vi "Get Scalar Datatypes and Refs.vi"(6 "Item Ref in":T1 format="%.0x", 8 "error in (no error)":errorcluster, 9 "Registers":T2[](array[typedef]) {"Register"."Data Type" format="%.0x"}, 10 "Data":dbl[](array[numeric]), 11 "Refs":T1[](array[typedef]) format="%.0x") -> (0 "error out":errorcluster, 1 "Registers out":T2[](array[typedef]) {"Register"."Data Type" format="%.0x"}, 2 "Data out":dbl[](array[numeric]), 3 "Refs out":T1[](array[typedef]) format="%.0x")   [LabVIEW 2018, in "FPGA Addon System Explorer.lvlib"]
uses:
  FPGA Addon System Explorer.lvlib
  Addon Shared/Types/Compiled.RegisterSettings.ctl
  Addon Shared/Types/Scalar Type.ctl
  Addon Shared/Types/Register Information.ctl
  Addon Shared/Types/FPGA Addon Data Type.ctl
  <vilib>/NI Veristand/Custom Device API/Custom Device Item Ref.ctl
  Addon Shared/Types/FG Action.ctl
  Addon Shared/SubVIs/Constants.vi
  <vilib>/NI/NI VeriStand Advanced SysDef API/SysDef API/SysDef.Property.Get.vi
  <vilib>/NI/NI VeriStand Advanced SysDef API/_SubVIs/SysDef.Property.Get.Variant.vi
  <vilib>/NI/NI VeriStand Advanced SysDef API/SysDef API/SysDef.Property.Set.vi
  <vilib>/NI/NI VeriStand Advanced SysDef API/_SubVIs/SysDef.Property.Set.Variant.vi
  <vilib>/NI Veristand/Custom Device API/Get Item Property (String).vi
  <vilib>/NI Veristand/Custom Device API/Custom Device API.lvlib
  Addon Shared/FPGA Addon Shared.lvlib
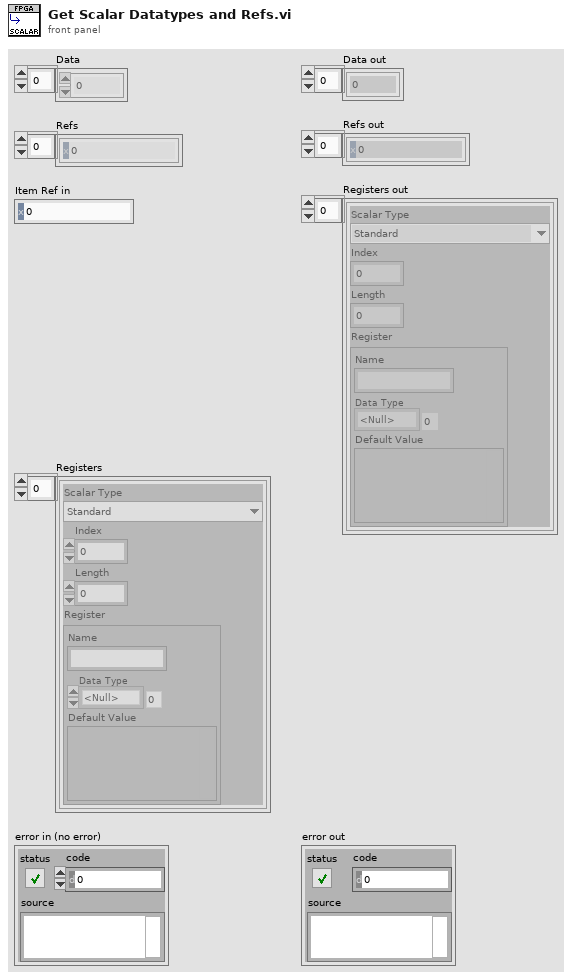
[diagram p1: front panel]
types:
  T1 = typedef "Custom Device API.lvlib/Custom Device Item Ref.ctl" = u64
  T2 = typedef "FPGA Addon Shared.lvlib/Compiled.RegisterSettings.ctl" = cluster{"Scalar Type":T3, "Index":i32, "Length":i32, "Register":T4}
  T3 = typedef "FPGA Addon Shared.lvlib/Scalar Type.ctl" = enum16{"Standard", "Bitpacked"}
  T4 = typedef "FPGA Addon Shared.lvlib/Register Information.ctl" = cluster{"Name":string, "Data Type":T5, "Default Value":variant}
  T5 = typedef "FPGA Addon Shared.lvlib/FPGA Addon Data Type.ctl" = enum8{"<Null>", "I8", "I16", "I32", "I64", "U8", "U16", "U32", "U64", "SGL", "Boolean", "Analog PWM In Settings", "Analog PWM In", "Digital PWM In Settings", "Digital PWM In", "Digital PWM Out", "Sine Out", "FXP", "FXP+/-24.5", "FXP+/-16.5", "FXP+/-32.8", "FXP+/-64.32", "FXP+/-16.7", "FXP+/-20.5", "FXP+/-27.5", "FXP+/-32.16", "FXP+16.3", "FXP+18.3", "Digital Static In", "Digital Static Out", "Digital Static In Settings", "Digital WSS Out", "Quad Encoder Settings", "Quad Encoder In", "Group"}
  T6 = typedef "FPGA Addon Shared.lvlib/FG Action.ctl" = enum8{"GET", "SET"}
  T7 = typedef "Custom Device API.lvlib/Custom Device Item Info.ctl" = cluster{"Name":string, "Is Channel":bool, "GUID":string, "Is Waveform":bool}
  T8 = typedef "Custom Device API.lvlib/Custom Device Channel.ctl" = cluster{"Type":T9, "Units":string, "Default Value":dbl, "Faultable":bool, "Scalable":bool}
  T9 = typedef "Custom Device API.lvlib/Custom Device Channel Type.ctl" = enum16{"Input", "Output"}
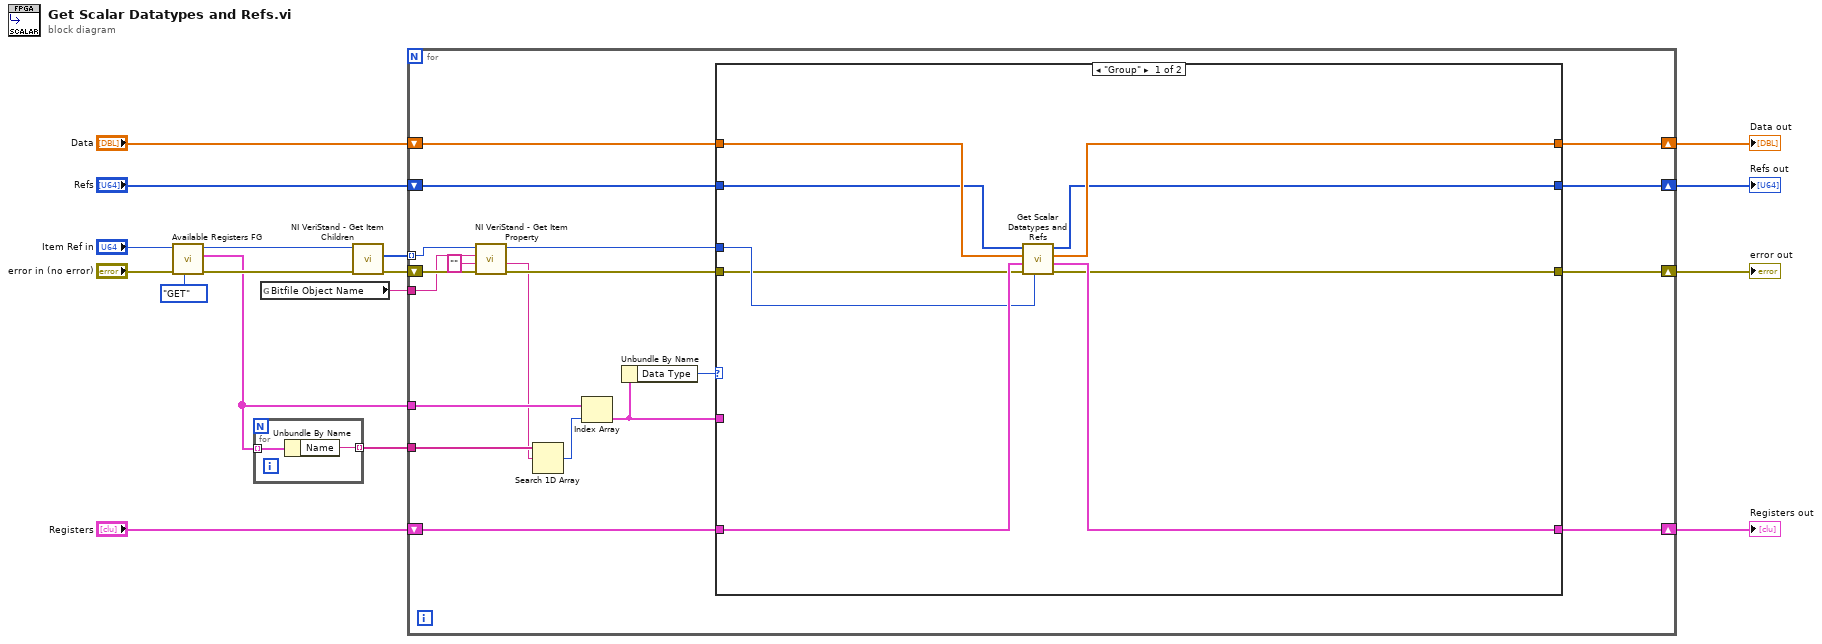
[diagram p0: block diagram]
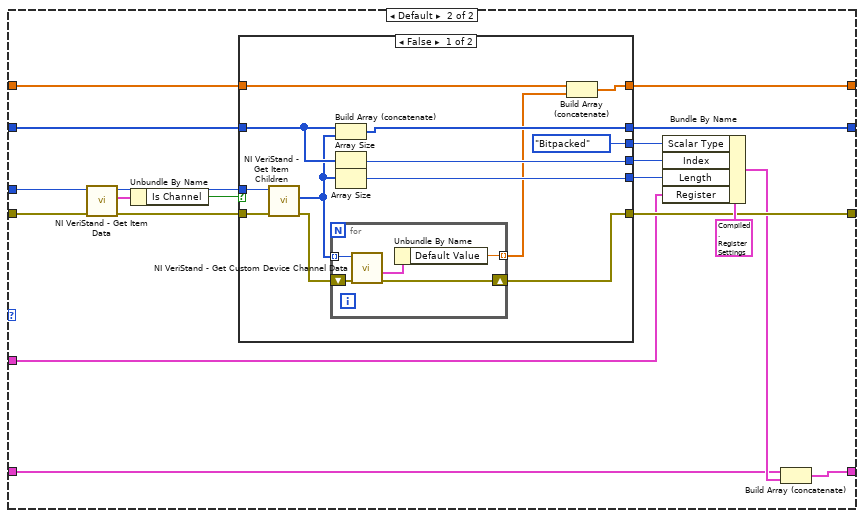
[diagram p2: hidden frame]
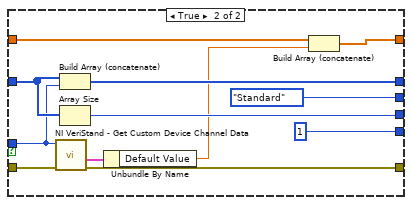
[diagram p3: hidden frame]
diagram:
  n1 = call "Available Registers FG.vi"("Action"=FG_Action."GET", "error in (no error)"="error in (no error)", "Item Ref"="Item Ref in") -> ("error out"=w4:errorcluster, "Available Registers"=w1:T4[], "Item Ref out"=w2:T1)  [unwired: 6 in]
  n2 = for {
    tunnel: w1 -> [w19] mode=indexing
    tunnel: [w18] -> w7 mode=indexing
    n3 = Unbundle By Name(w19) -> ("Name"=w18:string)
  }
  n4 = global read "Constants.vi" "Bitfile Object Name"() -> (w8:string)
  n5 = call <vilib>:"NI VeriStand - Get Item Children.vi"("error in (no error)"=w4, "Item Ref in"=w2) -> ("error out"=w10:errorcluster, "Child Refs"=w9:T1[])  [unwired: 6 in, 2 out]
  n6 = for {
    shift-right: [w26] -> w12
    shift-left: w10 -> [w38]
    tunnel: w9 -> [w37] mode=indexing
    tunnel: w8 -> [w36]
    tunnel: w7 -> [w34]
    tunnel: w1 -> [w32]
    shift-right: [w28] -> w13
    shift-left: "Refs" -> [w29]
    shift-right: [w25] -> w15
    shift-left: "Data" -> [w24]
    shift-right: [w22] -> w17
    shift-left: "Registers" -> [w21]
    n7 = call-poly <vilib>:"NI VeriStand - Get Item Property.vi"("error in (no error)"=w38, "Default Value"="", "Property Name"=w36, "Item Ref in"=w37) -> ("error out"=w30:errorcluster, "Value"=w27:string, "Item Ref out"=w33:T1)  [unwired: 4 in, 1 out]
    n8 = Search 1D Array(1D array=w34, element=w27) -> (index of element=w31:i32)  [unwired: 1 in]
    n9 = Index Array(array=w32, index=w31) -> (element=w23:T4)
    n10 = Unbundle By Name(w23) -> ("Data Type"=w20:T5)
    n11 = case shown="\"Group\"" w20 {
      tunnel: w33 -> [w41 w66]
      tunnel: w30 -> [w39 w65]
      tunnel: w29 -> [w46 w60]
      tunnel: [w44 w59] -> w28
      tunnel: [w40 w54] -> w26
      tunnel: [w45 w53] -> w25
      tunnel: w24 -> [w47 w52]
      tunnel: w23 -> [_ w51]
      tunnel: [w43 w49] -> w22
      tunnel: w21 -> [w42 w48]
      frame "Group" {
        n12 = call "Get Scalar Datatypes and Refs.vi"("Item Ref in"=w41, "error in (no error)"=w39, "Registers"=w42, "Data"=w47, "Refs"=w46) -> ("error out"=w40:errorcluster, "Registers out"=w43:T2[], "Data out"=w45:dbl[], "Refs out"=w44:T1[])  [unwired: 3 in]
      }
      frame Default {
        n13 = call <vilib>:"NI VeriStand - Get Item Data.vi"("error in (no error)"=w65, "Item Ref in"=w66) -> ("error out"=w62:errorcluster, "Item Info"=w64:T7, "Item Ref out"=w63:T1)  [unwired: 6 in, 1 out]
        n14 = Unbundle By Name(w64) -> ("Is Channel"=w61:bool)
        n15 = case shown="False" w61 {
          tunnel: w63 -> [w78 w91]
          tunnel: w62 -> [w79 w90]
          tunnel: [w69 w89] -> w54
          tunnel: w60 -> [w76 w94]
          tunnel: [w77 w96] -> w59
          tunnel: [Scalar_Type."Bitpacked" ("Scalar Type") Scalar_Type."Standard" ("Scalar Type")] -> w58
          tunnel: [w75 w93] -> w57
          tunnel: [w74 1] -> w56
          tunnel: [w67 w86] -> w53
          tunnel: w52 -> [w71 w85]
          frame False {
            n16 = call <vilib>:"NI VeriStand - Get Item Children.vi"("error in (no error)"=w79, "Item Ref in"=w78) -> ("error out"=w70:errorcluster, "Child Refs"=w72:T1[])  [unwired: 6 in, 2 out]
            n17 = for {
              tunnel: w72 -> [w83] mode=indexing
              shift-right: [w81] -> w69
              shift-left: w70 -> [w82]
              tunnel: [w80] -> w68 mode=indexing
              n18 = call <vilib>:"NI VeriStand - Get Custom Device Channel Data.vi"("error in (no error)"=w82, "Channel Ref in"=w83) -> ("error out"=w81:errorcluster, "Channel"=w84:T8)  [unwired: 4 in, 4 out]
              n19 = Unbundle By Name(w84) -> ("Default Value"=w80:dbl)
            }
            n20 = Build Array (concatenate)(w76, w72) -> (w77:T1[])
            n21 = Array Size(array=w76) -> (size(s)=w75:i32)
            n22 = Array Size(array=w72) -> (size(s)=w74:i32)
            n23 = Build Array (concatenate)(w71, w68) -> (w67:dbl[])
          }
          frame True {
            n24 = call <vilib>:"NI VeriStand - Get Custom Device Channel Data.vi"("error in (no error)"=w90, "Channel Ref in"=w91) -> ("error out"=w89:errorcluster, "Channel"=w88:T8)  [unwired: 4 in, 4 out]
            n25 = Build Array (concatenate)(w94, w91) -> (w96:T1[])
            n26 = Array Size(array=w94) -> (size(s)=w93:i32)
            n27 = Unbundle By Name(w88) -> ("Default Value"=w87:dbl)
            n28 = Build Array (concatenate)(w85, w87) -> (w86:dbl[])
          }
        }
        n29 = Bundle By Name(cluster=T2 {"Scalar Type"=enum."Standard", "Index"=0, "Length"=0, "Register"={"Name"="", "Data Type"=enum."<Null>", "Default Value"=variant(dbl 0.0)}} ("Cluster"), "Scalar Type"=w58, "Index"=w57, "Length"=w56, "Register"=w51) -> (w50:T2)
        n30 = Build Array (concatenate)(w48, w50) -> (w49:T2[])
      }
    }
  }
  "Registers out" <- w17
  "Data out" <- w15
  "Refs out" <- w13
  "error out" <- w12
